vi "Convert Path To Array Of Folders.vi"(1 "Folder Path":path) -> (0 "Individual Folders":string[](array[string]))   [LabVIEW 2022 SP3]
doc: "This VI takes a Folder Path and returns an array of individual folder names as output. Array index 0 is the root folder.\n\nExample 1\nFolder Path = \"C:\\Power Supply Library\"\nIndividual Folders = \"[C] [Power Supply Library]\"\n\nExample 2\nFolder Path = \"C:\\Power Supply Library\\Basic Functions\"\nIndividual Folders = \"[C] [Power Supply Library] [Basic Functions]\"\n\nExample 3\nFolder Path = \"C:\\abc\\def\\ghi\\jkl\"\nIndividual Folders = \"[C] [abc] [def] [ghi] [jkl]\""
panel:
  out "Iteration":i32
  # "Development\nControls or indicators that are useful for development or testing, but which are not outputs of the VI."
  # "Input\nInputs to the VI"
  # "Output\nOutputs of the VI"
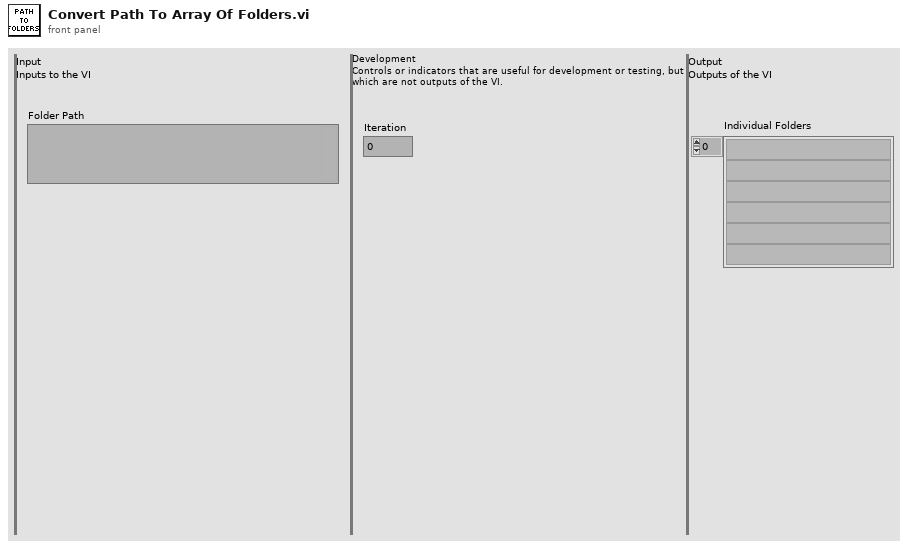
[diagram p1: front panel]
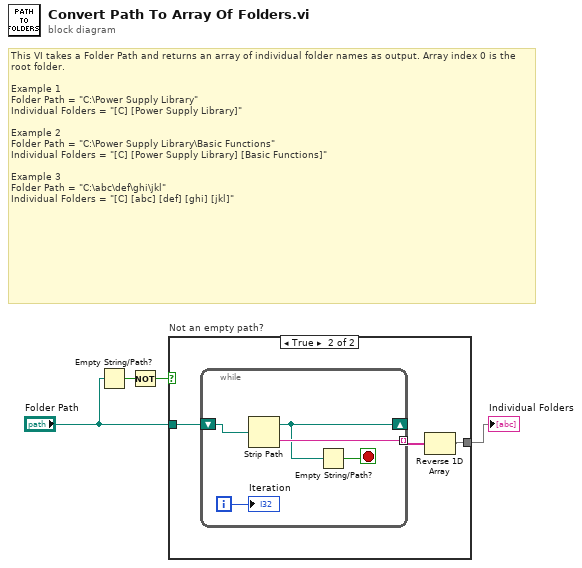
[diagram p0: block diagram]
diagram:
  # "This VI takes a Folder Path and returns an array of individual folder names as output. Array index 0 is the root folder.\n\nExample 1\nFolder Path = \"C:\\Power Supply Library\"\nIndividual Folders = \"[C] [Power Supply Library]\"\n\nExample 2\nFolder Path = \"C:\\Power Supply Library\\Basic Functions\"\nIndividual Folders = \"[C] [Power Supply Library] [Basic Functions]\"\n\nExample 3\nFolder Path = \"C:\\abc\\def\\ghi\\jkl\"\nIndividual Folders = \"[C] [abc] [def] [ghi] [jkl]\""
  n1 = Empty String/Path?(string/path="Folder Path") -> (empty?=w4:bool)
  n2 = Not(x=w4) -> (.not. x?=w3:bool)
  n3 = case "Not an empty path?" shown="True" w3 {
    tunnel: "Folder Path" -> [_ w7]
    tunnel: [_ w5] -> w1
    frame False {
      # "Empty path in. \nReturn empty array."
    }
    frame True {
      n4 = while {
        shift-right: [w9] -> _
        shift-left: w7 -> [w12]
        tunnel: [w11] -> w6 mode=indexing
        i -> [w8]
        stop <- w10 stop-if-true
        n5 = Strip Path(path=w12) -> (stripped path=w9:path, name=w11:string)
        n6 = Empty String/Path?(string/path=w9) -> (empty?=w10:bool)
        "Iteration" <- w8
      }
      n7 = Reverse 1D Array(array=w6) -> (reversed array=w5:string[])
    }
  }
  "Individual Folders" <- w1
